vi "Set Created.vi"(10 "Created":T1, 11 "Addresses in":refnum<class "Addresses.lvclass">) -> (3 "Addresses out":refnum<class "Addresses.lvclass">)   [LabVIEW 2021, in "jettl.lvlib" / "Addresses.lvlib" / "Addresses.lvclass"]
uses:
  Addresses.lvclass
  Addresses.lvclass/Addresses.ctl
  Msg Type Strategy/Msg Type Strategy/Msg Type Strategy.lvclass
  Created.ctl
  Addresses.lvlib
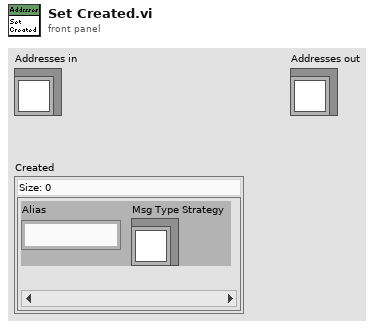
[diagram p1: front panel]
types:
  T1 = typedef "jettl.lvlib/Addresses.lvlib/Created.ctl" = map{string, refnum<class "Msg Type Strategy.lvclass">}
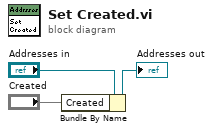
[diagram p0: block diagram]
diagram:
  n1 = Bundle By Name(cluster="Addresses in", "Created"="Created") -> (→"Addresses out":refnum<class "Addresses.lvclass">)
